vi "Status Created Queues.vi"(11 "Hello World Event in":refnum<class "Hello World Event.lvclass">) -> (0 "Created Queue Count":i32, 1 "Created Queue Aliases":string[](array[string]), 2 "Created Queue Exist?":bool, 3 "Hello World Event out":refnum<class "Hello World Event.lvclass">)   [LabVIEW 2021, in "Hello World Event.lvlib" / "Hello World Event.lvclass"]
uses:
  Hello World Event.lvclass
  Hello World Event.lvclass/Hello World Event.ctl
  jettl/Event jettl/Event jettl.lvclass
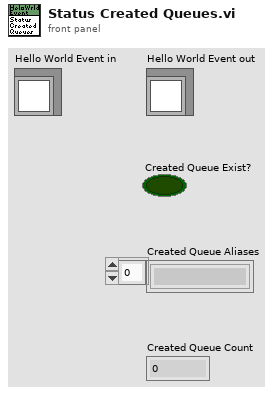
[diagram p1: front panel]
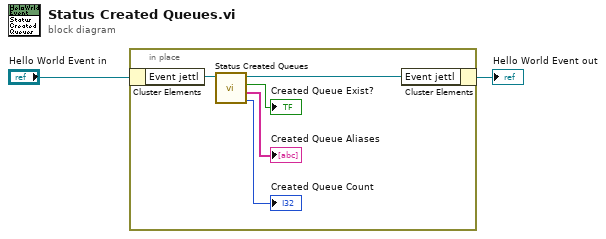
[diagram p0: block diagram]
diagram:
  n1 = in-place {
    n2 = in-place-cluster #1("Hello World Event in") -> ("Event jettl"=w7:refnum<class "Event jettl.lvclass">)
    n3 = call-dynamic "Status Created Queues.vi"("jettl in"=w7) -> ("Created Queue Count"=→"Created Queue Count":i32, "Created Queue Aliases"=→"Created Queue Aliases":string[], "Created Queue Exist?"=→"Created Queue Exist?":bool, "jettl out"=w6:refnum<class "Event jettl.lvclass">)  [unwired: 7 in]
    n4 = in-place-cluster #1("Event jettl"=w6) -> (→"Hello World Event out":refnum<class "Hello World Event.lvclass">)
  }
